vi "wave pulse generator (SubVI).vi"(0 "VISA Refnum in":refnum<visa-resource-name>, 1 "Amplitude (1.0 Vpp)":dbl=1.0 format="%#.3f", 2 "Waveform Function (0: Sine) in":u16(ring) items=["Sine", "Square", "Ramp", "DC", "Pulse", "Arb"], 3 "Enable Output (T: Enable)":bool=TRUE, 4 "True To \ngenerate\n pulse":bool, 5 "error in (no error)":errorcluster, 6 "Channel (1:Channel 1)":i32(ring)=1 items=["Channel 1"=1, "Channel 2"=2], 7 "Frequency (1000 Hz)":dbl=1000.0 format="%#.6g", 8 "Rise (20 ns)":dbl=2e-08 format="%#.3g", 9 "DC Offset (0.00 V) in":dbl, 10 "Delay (0.00 s)":dbl min=-1000000.0 max=1000000.0, 11 "Phase (0.0 degrees)":dbl=0.002 min=-360.0 max=360.0 format="%#.1g", 12 "Duty (20%)":dbl=20.0 min=0.0001 max=100.0 format="%.4g", 13 "Fall (20 ns)":dbl=2e-08 format="%#.3g") -> (14 "VISA Refnum out":refnum<visa-resource-name>, 19 "error out":errorcluster)   [LabVIEW 2018, in "Siglent SDG X Series.lvlib"]
uses:
  <instrlib>/Siglent SDG X Series/Siglent SDG X Series.lvlib
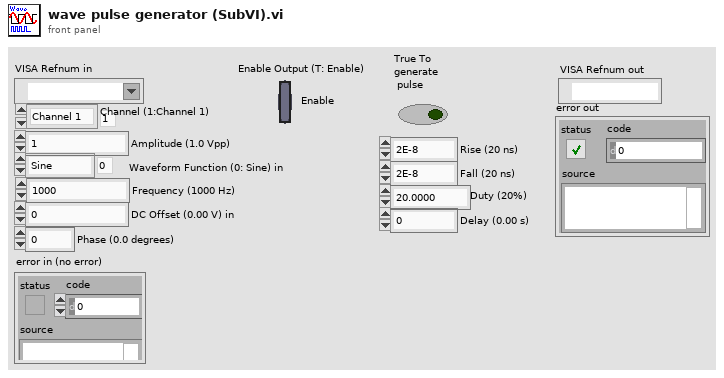
[diagram p1: front panel]
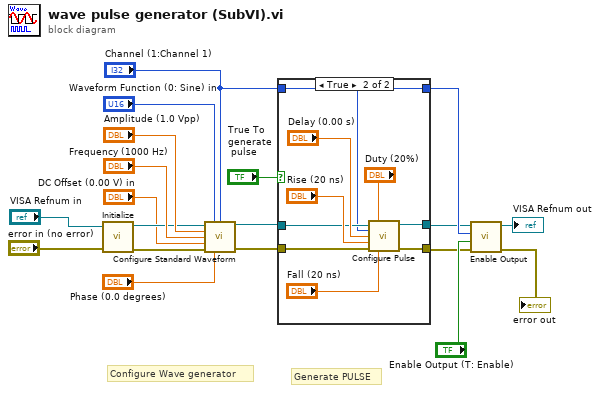
[diagram p0: block diagram]
diagram:
  # "Configure Wave generator"
  # "Generate PULSE"
  n1 = call <instrlib>:"Initialize.vi"("error in (no error)"="error in (no error)", "VISA resource name"="VISA Refnum in") -> ("error out"=w8:errorcluster, "VISA resource name out"=w7:refnum<visa-resource-name>)  [unwired: 8 in]
  n2 = call <instrlib>:"Configure Standard Waveform.vi"("VISA resource name"=w7, "Waveform Function (0: Sine)"="Waveform Function (0: Sine) in", "Channel (1:Channel 1)"="Channel (1:Channel 1)", "Amplitude (1.0 Vpp)"="Amplitude (1.0 Vpp)", "Frequency (1000 Hz)"="Frequency (1000 Hz)", "DC Offset (0.00 V)"="DC Offset (0.00 V) in", "error in (no error)"=w8, "Phase (0.0 degrees)"="Phase (0.0 degrees)") -> ("VISA resource name out"=w14:refnum<visa-resource-name>, "error out"=w9:errorcluster)  [unwired: 6 in]
  n3 = case shown="True" "True To \ngenerate\n pulse" {
    tunnel: [w20 w25] -> w2
    tunnel: [w19 w24] -> w3
    tunnel: w14 -> [w20 w23]
    tunnel: w9 -> [w19 w22]
    tunnel: "Channel (1:Channel 1)" -> [_ w21]
    tunnel: "Channel (1:Channel 1)" -> [_ _]
    frame False {
    }
    frame True {
      n4 = call <instrlib>:"Configure Pulse.vi"("VISA resource name"=w23, "Duty (20%)"="Duty (20%)", "Channel (1:Channel 1)"=w21, "Delay (0.00 s)"="Delay (0.00 s)", "Rise (20 ns)"="Rise (20 ns)", "error in (no error)"=w22, "Fall (20 ns)"="Fall (20 ns)") -> ("VISA resource name out"=w25:refnum<visa-resource-name>, "error out"=w24:errorcluster)  [unwired: 7 in]
    }
  }
  n5 = call <instrlib>:"Enable Output.vi"("error in (no error)"=w3, "Enable Output (T: Enable)"="Enable Output (T: Enable)", "Channel (1:Channel 1)"="Channel (1:Channel 1)", "VISA resource name"=w2) -> ("error out"=→"error out":errorcluster, "VISA resource name out"=→"VISA Refnum out":refnum<visa-resource-name>)  [unwired: 6 in]
